vi "DAC Init Results.vi"(8 "error in":errorcluster, 9 "Log Details?":bool, 10 "tdms file":refnum<k34>, 11 "DAC in":refnum<class "DAC.lvclass">) -> (0 "error out":errorcluster, 2 "tdms file out":refnum<k34>)   [LabVIEW 2019, in "DAC.lvlib" / "DAC.lvclass"]
uses:
  DAC.lvclass
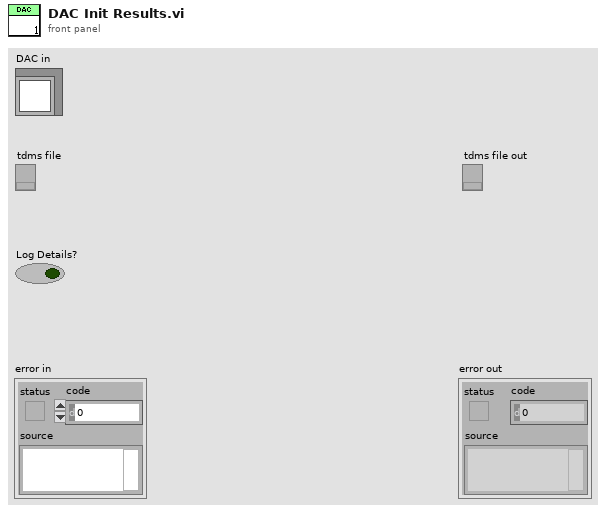
[diagram p1: front panel]
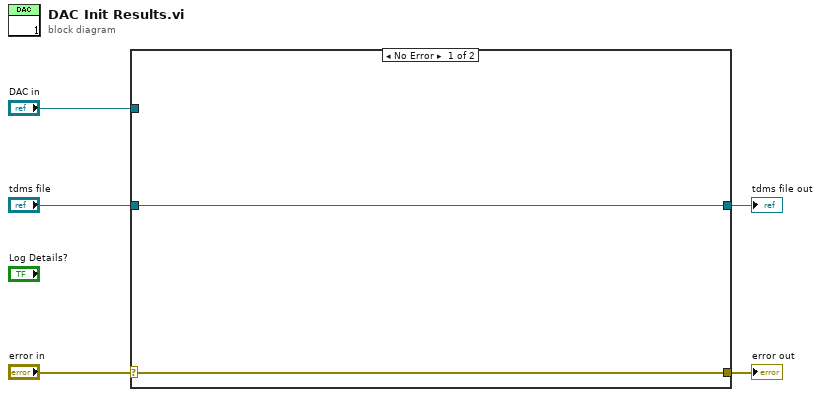
[diagram p0: block diagram]
diagram:
  n1 = case shown="No Error" "error in" {
    selector: "error in" -> [w7 w9]
    tunnel: [w7 w9] -> w4
    tunnel: "DAC in" -> [_ _]
    tunnel: "tdms file" -> [w6 w8]
    tunnel: [w6 w8] -> w1
    frame No Error {
    }
    frame Error {
    }
  }
  "error out" <- w4
  "tdms file out" <- w1
